vi "Three devices step test.vi"() -> ()   [LabVIEW 2015]
doc: "This example VI shows how to convert string data elements to numeric elements so it can be graphed and displayed on an XY Graph."
uses:
  <instrlib>/Keithley 27XX/Public/Configure/Measurement Specific/Configure Thermocouple.vi
  <instrlib>/Ke24xx/Ke24xx.llb/Ke24xx Configure Source Volt/Cur Level.vi
  <instrlib>/Ke24xx/Ke24xx.llb/Ke24xx Enable/Disable Source Output.vi
  <instrlib>/Keithley 27XX/Keithley 27XX.lvlib
panel:
  in  "level":dbl min=-1100.0 max=1100.0 step=1.0 format="%.2p"
  in  "Compliance":dbl=1.0 min=-1100.0 max=1100.0 step=1.0 format="%.2p"
  out "error out Cryocon":errorcluster
  out "error out 2425":errorcluster
  in  "Loop 2":bool
  in  "range":i32
  in  "function":i32(slide)
  in  "error in (no error) 2":errorcluster
  in  "reset device":u16(slide)=1
  in  "id query":u16(slide)=1
  in  "resource name":string="GPIB0::20::INSTR"
  out "Delta":dbl
  out "Variance":string
  in  "Setpoint (K)":dbl=300.0
  in  "D":sgl format="%.2f"
  in  "I":sgl=30.0 min=0 step=1 format="%.2f"
  in  "P":sgl=5.0 format="%.2f"
  in  "Output":u8(ring) items=["Loop 1", "Loop 2"]
  in  "Loop 1":bool
  out "Minimum":string
  out "Time Since Reset (Mins)":string
  out "Maximum":string
  out "Offset":string
  out "Cryocon Temp":dbl(graph)
  in  "Set Input":u8(ring) items=["ChA", "ChB", "ChC", "ChD"]
  in  "error in (no error)":errorcluster
  in  "baud rate (9600)":u32=9600
  in  "Port":string="10::INSTR"
  in  "Interface":u16(ring) items=["GPIB", "Serial"]
  in  "Save File?":bool
  out "Channel 3":dbl[](graph)
  out "Channel 2":dbl[](graph)
  out "Channel 1":dbl[](graph)
  in  "Enable Open Detector? (False)":bool
  in  "Simulated Reference Temperature (23 deg C)":dbl=23.0
  in  "Reference Junction Type (0: Simulated)":u16(ring)=1 items=["Simulated", "Internal", "External"]
  in  "Thermocouple Type (1: K)":u16(ring)=1 items=["J", "K", "T", "E", "R", "S", "B", "N"]
  in  "Column headers":string[](array[string])=["Time/s", "Cryocon Temp/C", "Ch101 Temp/C", "", "", "", ""]
  in  "Number of channels":i32=1
  in  "Pause/Continue":bool
  in  "stop":bool
  out "Iterations":i32
  out "concatenated string":string
  in  "file (use dialog)":path=path "C:/Users/Guest_2/Desktop/Zong Long/Data trial.txt"
  in  "Function (6: Temp)":u16(ring)=6 items=["DC Voltage", "AC Voltage", "DC Current", "AC Current", "Resistance", "Four-Wire Resistance", "Temperature (C)", "Frequency", "Period", "Continuity"]
  in  "Channel List (101)":string="101"
  in  "Serial Configuration":T1={"Baud Rate (9600)"=9600, "Flow Control (1: XON/XOFF)"=1, "Termination Char (0:CR)"=0} {"Termination Char (0:CR)" items=["CR", "LF", "CRLF (Do not use)", "LFCR (Do not use)"]; "Flow Control (1: XON/XOFF)" items=["None", "XON/XOFF", "RTS/CTS (2701 Only)", "XON/XOFF & RTS/CTS (2701 Only)"]; "Baud Rate (9600)" items=["300"=300, "600"=600, "1200"=1200, "2400"=2400, "4800"=4800, "9600"=9600, "19.2k"=19200, "38.4k (2701 Only)"=38400, "57.6k (2701 Only)"=57600, "115.2k (2701 Only)"=115200]}
  in  "Keithley VISA \nresource name":refnum<visa-resource-name>="GPIB0::19::INSTR"
  # "Keithley 2425 INIT"
  # "Cryocon INIT"
  # "File INIT"
  # "Keithley 2700 INIT"
  # "Operations"
  # "Only Loop 1 implemened"
  # "Data"
  # "Loop 1"
  # "Loop 2"
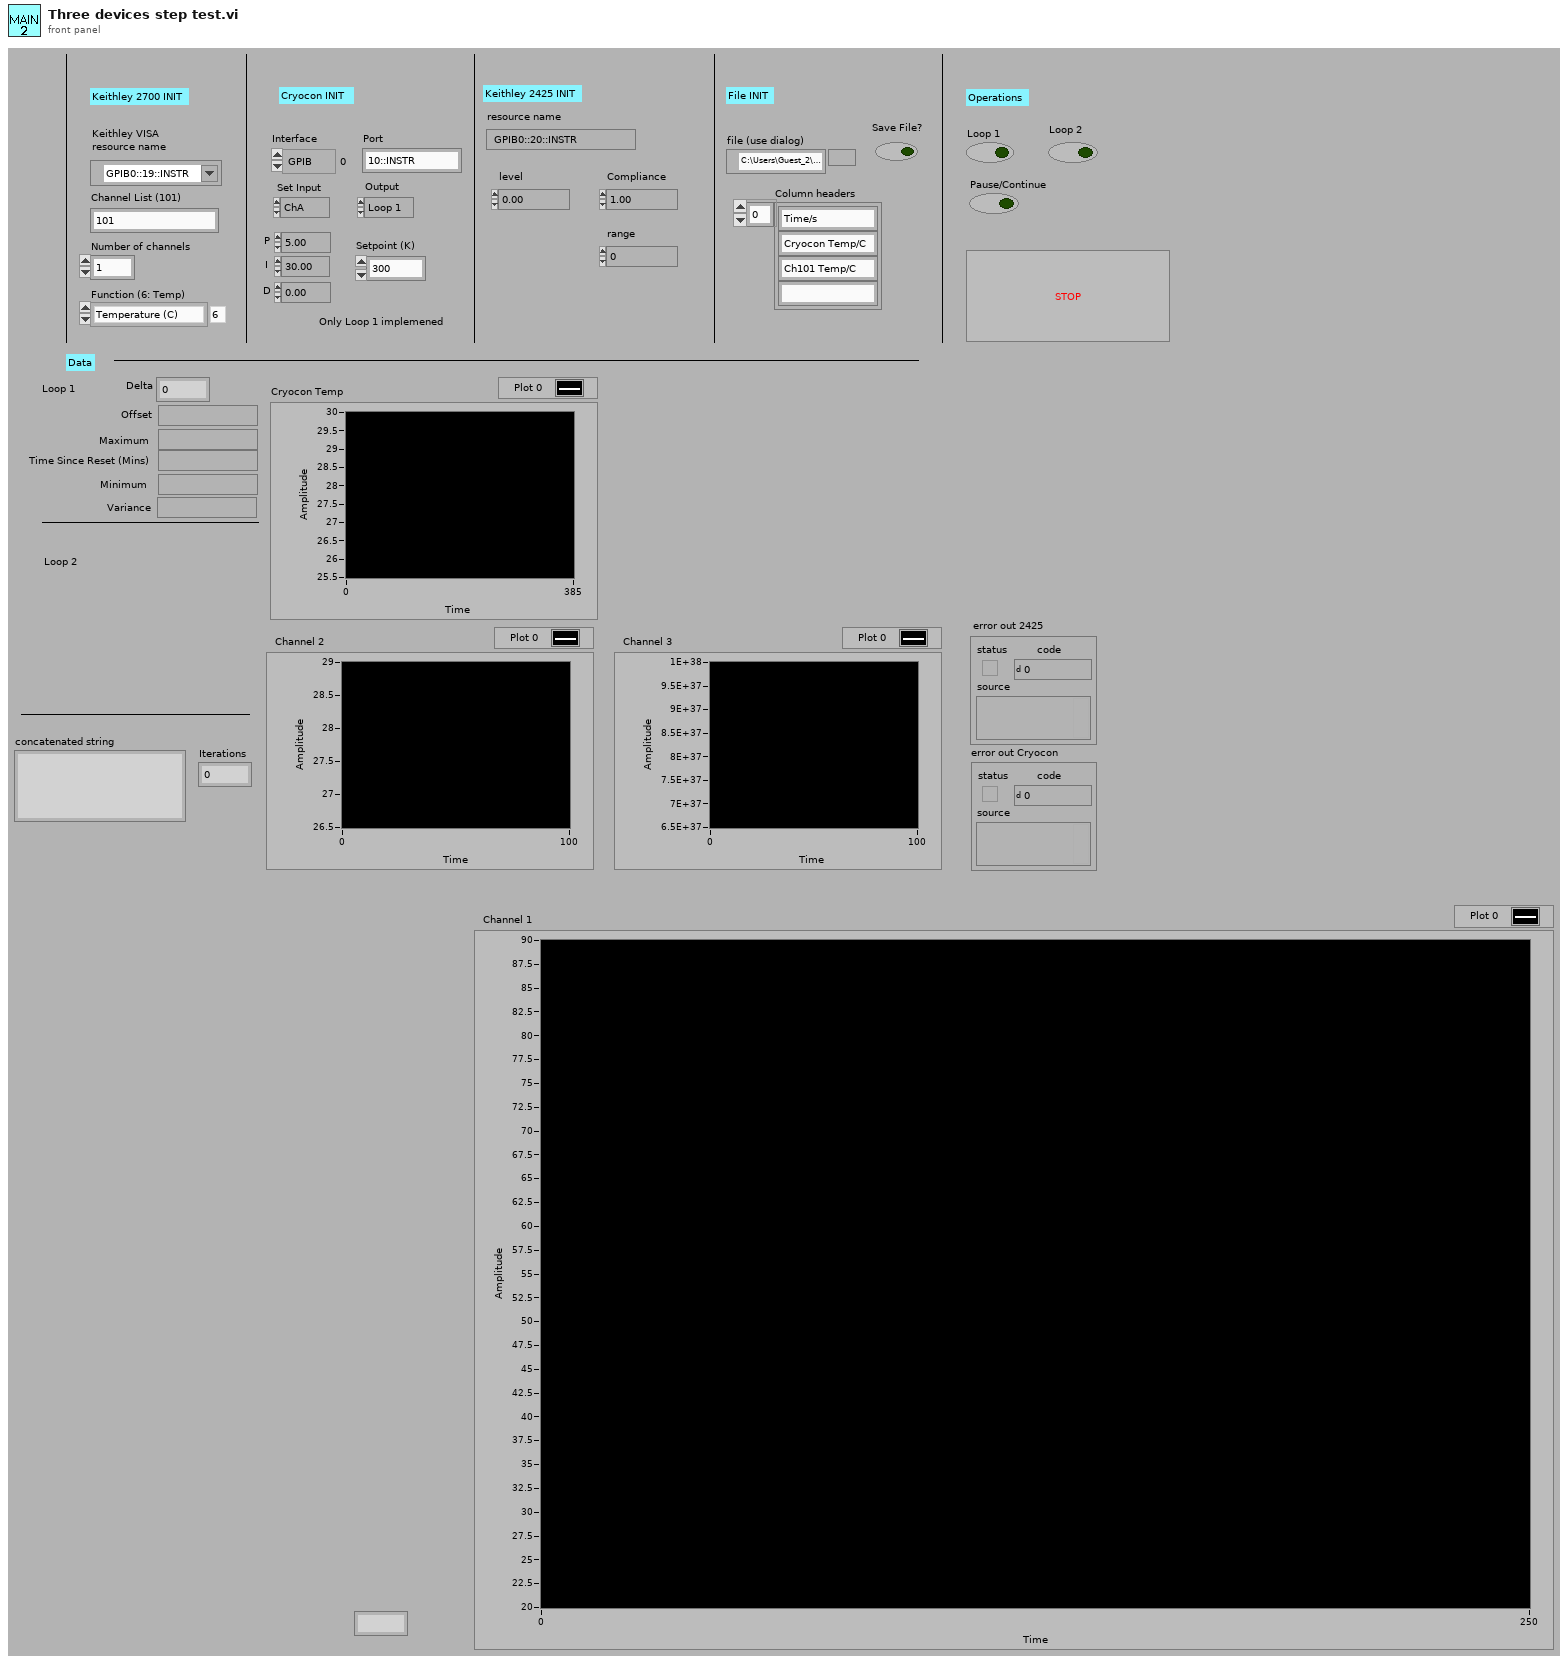
[diagram p1: front panel]
types:
  T1 = cluster{"Baud Rate (9600)":u32, "Flow Control (1: XON/XOFF)":u16, "Termination Char (0:CR)":u16}
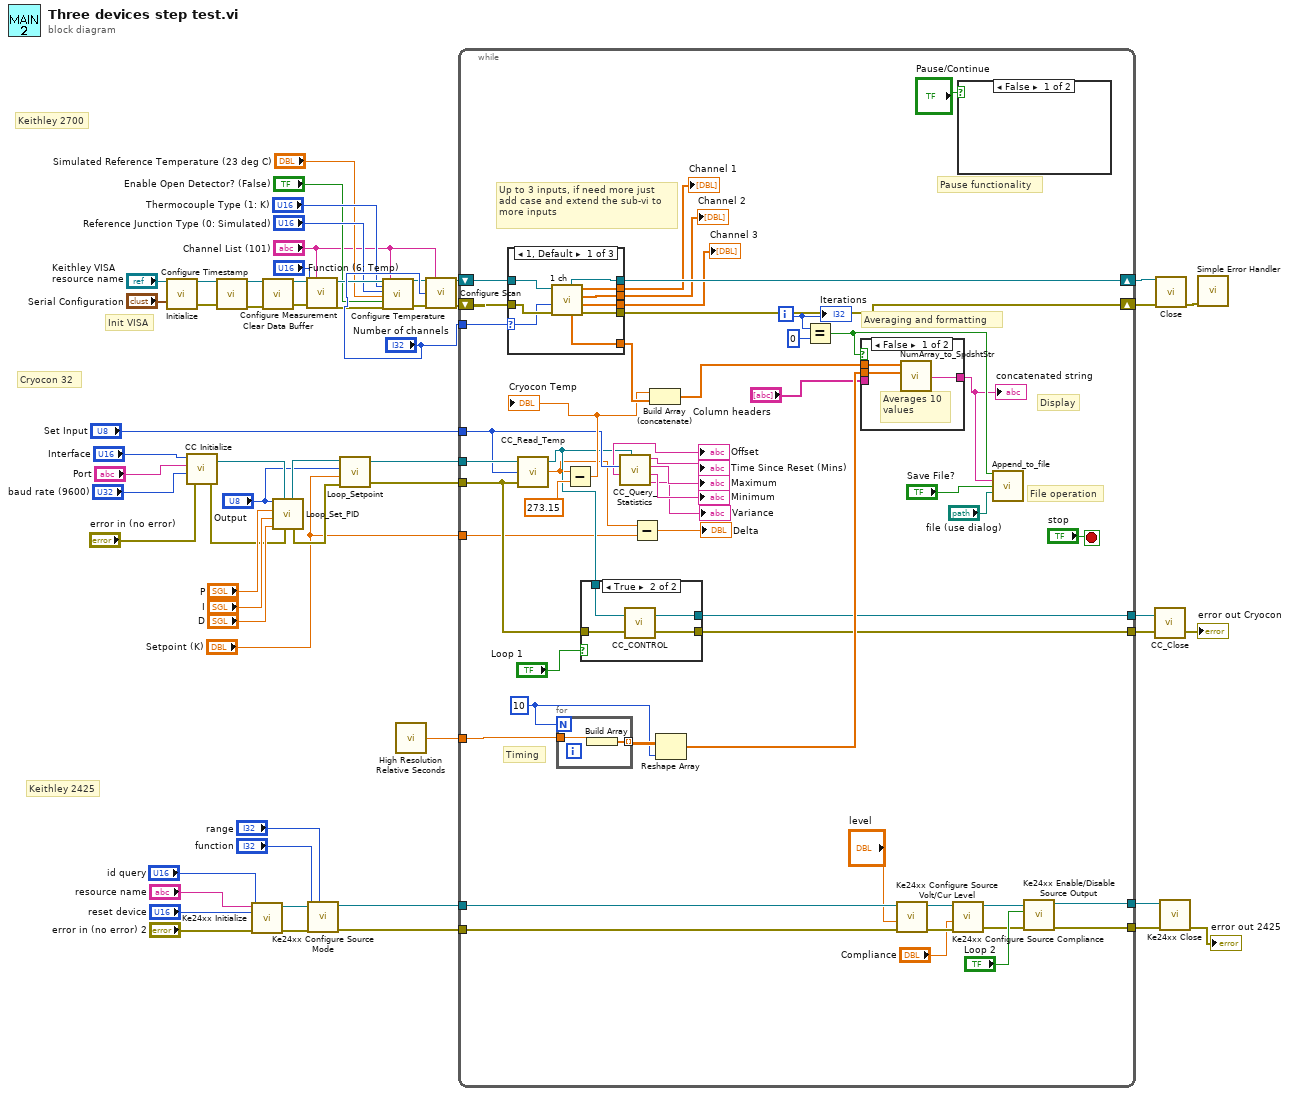
[diagram p0: block diagram]
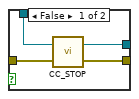
[diagram p2: hidden frame]
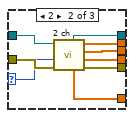
[diagram p3: hidden frame]
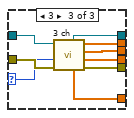
[diagram p4: hidden frame]
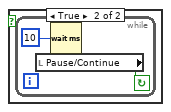
[diagram p5: hidden frame]
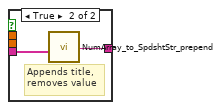
[diagram p6: hidden frame]
diagram:
  # "Keithley 2425"
  # "Cryocon 32"
  # "Keithley 2700"
  # "Init VISA"
  n1 = call <instrlib>:"Initialize.vi"("VISA resource name"="Keithley VISA \nresource name", "Serial Configuration"="Serial Configuration") -> ("VISA resource name out"=w54:refnum<visa-resource-name>, "error out"=w53:errorcluster)  [unwired: 12 in]
  n2 = call "CC Initialize.vi"("error in (no error)"="error in (no error)", "baud rate (9600)"="baud rate (9600)", "Port"="Port", "Interface"="Interface") -> ("error out"=w22:errorcluster, "VISA out"=w21:refnum<visa-resource-name>)
  n3 = call <instrlib>:"Configure Timestamp.vi"("VISA resource name"=w54, "error in (no error)"=w53) -> ("VISA resource name out"=w49:refnum<visa-resource-name>, "error out"=w48:errorcluster)  [unwired: 12 in]
  n4 = call <instrlib>:"Ke24xx Initialize.vi"("error in (no error)"="error in (no error) 2", "reset device"="reset device", "id query"="id query", "resource name"="resource name") -> ("error out"=w9:errorcluster, "instrument handle out"=w10:refnum<visa-resource-name>)  [unwired: 5 in, 1 out]
  n5 = call <instrlib>:"Clear Data Buffer.vi"("VISA resource name"=w49, "error in (no error)"=w48) -> ("VISA resource name out"=w47:refnum<visa-resource-name>, "error out"=w50:errorcluster)  [unwired: 12 in]
  n6 = call "Loop_Set_PID"("error in (no error)"=w22, "VISA In"=w21, "D"="D", "I"="I", "P"="P", "Output"="Output") -> ("error out"=w20:errorcluster, "VISA Out"=w19:refnum<visa-resource-name>)  [unwired: 4 in]
  n7 = call <instrlib>:"Configure Measurement.vi"("VISA resource name"=w47, "Scan List (Empty)"="Channel List (101)", "Function (0: DC Voltage)"="Function (6: Temp)", "error in (no error)"=w50) -> ("VISA resource name out"=w41:refnum<visa-resource-name>, "error out"=w38:errorcluster)  [unwired: 10 in]
  n8 = call <instrlib>:"Ke24xx Configure Source Mode.vi"("range"="range", "error in (no error)"=w9, "function"="function", "instrument handle"=w10) -> ("error out"=w1:errorcluster, "instrument handle out"=w2:refnum<visa-resource-name>)  [unwired: 5 in, 1 out]
  n9 = call "Loop_Setpoint.vi"("VISA in"=w19, "Loop"="Output", "Setpoint"="Setpoint (K)", "error in"=w20) -> ("VISA out"=w18:refnum<visa-resource-name>, "ErrorOut"=w16:errorcluster)  [unwired: 1 in, 1 out]
  n10 = call-poly <instrlib>:"Configure Temperature.vi"("VISA resource name"=w41, "Thermocouple Type (1: K)"="Thermocouple Type (1: K)", "Reference Junction Type (0: Simulated)"="Reference Junction Type (0: Simulated)", "Simulated Reference Temperature (23 deg C)"="Simulated Reference Temperature (23 deg C)", "Enable Open Detector? (False)"="Enable Open Detector? (False)", "error in (no error)"=w38, "Scan List (Empty)"="Channel List (101)") -> ("VISA resource name out"=w40:refnum<visa-resource-name>, "error out"=w39:errorcluster)  [unwired: 11 in]
  n11 = call <vilib>:"High Resolution Relative Seconds.vi"() -> ("relative seconds"=w43:dbl)
  n12 = call <instrlib>:"Configure Scan.vi"("VISA resource name"=w40, "Channel List (101:110)"="Channel List (101)", "Sample Count (100)"="Number of channels", "error in (no error)"=w39) -> ("VISA resource name out"=w45:refnum<visa-resource-name>, "error out"=w44:errorcluster)  [unwired: 10 in]
  n13 = while {
    shift-right: [w107] -> w51
    shift-left: w45 -> [w106]
    shift-right: [w108] -> w52
    shift-left: w44 -> [w105]
    tunnel: w43 -> [w103]
    tunnel: "Number of channels" -> [w96]
    tunnel: "Set Input" -> [w83]
    tunnel: w18 -> [w88]
    tunnel: w16 -> [w76]
    tunnel: [w75] -> w27
    tunnel: [w74] -> w26
    tunnel: "Setpoint (K)" -> [w71]
    tunnel: [w68] -> w6
    tunnel: [w67] -> w5
    tunnel: w2 -> [w66]
    tunnel: w1 -> [w65]
    i -> [w98]
    stop <- "stop" stop-if-true
    w95 = 10 ("x")
    # "Timing"
    # "Up to 3 inputs, if need more just\nadd case and extend the sub-vi to\nmore inputs"
    # "Display"
    # "Averaging and formatting"
    # "File operation"
    # "Pause functionality"
    n14 = case shown="1, Default" w96 {
      selector: w96 -> [w124 w131 w140]
      tunnel: [w120 w132 w141] -> w108
      tunnel: [w122 w129 w139] -> w107
      tunnel: w106 -> [w123 w134 w142]
      tunnel: w105 -> [w125 w133 w143]
      tunnel: [w119 w127 w137] -> w59
      tunnel: [w118 w128 w136] -> w94
      tunnel: [w117 w130 w135] -> w93
      tunnel: [w121 w126 w138] -> w86
      frame 1, Default {
        n15 = call "1 ch.vi"("error out"=w125, "Number of channels"=w124, "VISA resource name out"=w123) -> ("error out 2"=w120:errorcluster, "output array 3"=w117:dbl[], "output array 2"=w118:dbl[], "Means of 10"=w119:dbl[], "output array"=w121:dbl[], "VISA resource name out 2"=w122:refnum<visa-resource-name>)  [unwired: 3 in]
      }
      frame 2 {
        n16 = call "2 ch.vi"("error out"=w133, "Number of channels"=w131, "VISA resource name out"=w134) -> ("error out 2"=w132:errorcluster, "Means of 12"=w130:dbl[], "Means of 11"=w128:dbl[], "Means of 10"=w127:dbl[], "output array"=w126:dbl[], "VISA resource name out 2"=w129:refnum<visa-resource-name>)  [unwired: 3 in]
      }
      frame 3 {
        n17 = call "3 ch.vi"("error out"=w143, "Number of channels"=w140, "VISA resource name out"=w142) -> ("error out 2"=w141:errorcluster, "Means of 12"=w135:dbl[], "Means of 11"=w136:dbl[], "Means of 10"=w137:dbl[], "output array"=w138:dbl[], "VISA resource name out 2"=w139:refnum<visa-resource-name>)  [unwired: 3 in]
      }
    }
    "Channel 3" <- w93
    "Channel 2" <- w94
    "Channel 1" <- w59
    n18 = call "CC_Read_Temp.vi"("error in (no error)"=w76, "Input"=w83, "VISA In"=w88) -> ("Temperature"=w72:dbl, "VISA Out"=w77:refnum<visa-resource-name>)  [unwired: 1 out]
    n19 = for {
      N: w95 -> [_]
      tunnel: w103 -> [w147]
      tunnel: [w146] -> w102 mode=indexing
      n20 = Build Array(w147) -> (w146:dbl[])
    }
    n21 = Subtract(x=w72, y=273.15) -> (x-y=w84:dbl)
    "Cryocon Temp" <- w84
    n22 = case shown="True" "Loop 1" {
      tunnel: w77 -> [w112 w116]
      tunnel: w76 -> [w111 w115]
      tunnel: [w110 w114] -> w75
      tunnel: [w109 w113] -> w74
      frame False {
        n23 = call "CC_STOP.vi"("error in (no error)"=w111, "VISA In"=w112) -> ("error out"=w109:errorcluster, "VISA Out"=w110:refnum<visa-resource-name>)
      }
      frame True {
        n24 = call "CC_CONTROL.vi"("error in (no error)"=w115, "VISA In"=w116) -> ("error out"=w113:errorcluster, "VISA Out"=w114:refnum<visa-resource-name>)
      }
    }
    n25 = call "CC_Query_Statistics.vi"("VISA In"=w77, "Input"=w83) -> ("Variance"=→"Variance":string, "Minimum"=→"Minimum":string, "Maximum"=→"Maximum":string, "Time Since Reset"=→"Time Since Reset (Mins)":string, "Offset"=→"Offset":string)  [unwired: 2 in, 3 out]
    n26 = Subtract(x=w72, y=w71) -> (x-y=→"Delta":dbl)
    n27 = Build Array (concatenate)(w84, w86) -> (w87:dbl[])
    n28 = Reshape Array(w102, w95) -> (w101:dbl[])
    n29 = Equal?(x=w98, y=0) -> (x = y?=w91:bool)
    n30 = case shown="False" w91 {
      tunnel: w87 -> [w150 _]
      tunnel: w101 -> [w149 _]
      tunnel: [w148 w152] -> w90
      tunnel: "Column headers" -> [_ w151]
      frame False {
        # "Averages 10 \nvalues"
        n31 = call "NumArray_to_SpdshtStr.vi"("element 2"=w149, "element"=w150) -> ("concatenated string"=w148:string)  [unwired: 8 in, 1 out]
      }
      frame True {
        # "Appends title,\nremoves value"
        n32 = call "NumArray_to_SpdshtStr_prepend.vi"("Column headers"=w151) -> ("concatenated string"=w152:string)  [unwired: 10 in]
      }
    }
    "concatenated string" <- w90
    n33 = call "Ke24xx Configure Source Volt/Cur Level.vi"("error in (no error)"=w65, "level"="level", "instrument handle"=w66) -> ("error out"=w63:errorcluster, "instrument handle out"=w64:refnum<visa-resource-name>)  [unwired: 6 in, 1 out]
    n34 = call <instrlib>:"Ke24xx Configure Source Compliance.vi"("error in (no error)"=w63, "level"="Compliance", "instrument handle"=w64) -> ("error out"=w61:errorcluster, "instrument handle out"=w62:refnum<visa-resource-name>)  [unwired: 6 in, 1 out]
    n35 = case shown="False" "Pause/Continue" {
      frame False {
      }
      frame True {
        n36 = while {
          stop <- w145 continue-if-true
          n37 = local read "Pause/Continue"() -> (w145:bool)
          n38 = Wait (ms)(milliseconds to wait=u32 10) -> ()  [unwired: 1 out]
        }
      }
    }
    n39 = call "Append_to_file.vi"("Boolean"=w91, "text"=w90, "Save File?"="Save File?", "file path (use dialog)"="file (use dialog)") -> ()  [unwired: 11 in, 1 out]
    n40 = call "Ke24xx Enable/Disable Source Output.vi"("error in (no error)"=w61, "state"="Loop 2", "instrument handle"=w62) -> ("error out"=w67:errorcluster, "instrument handle out"=w68:refnum<visa-resource-name>)  [unwired: 6 in, 1 out]
    "Iterations" <- w98
  }
  n41 = call "CC_Close.vi"("error in (no error)"=w26, "VISA In"=w27) -> ("error out"=→"error out Cryocon":errorcluster)  [unwired: 1 in]
  n42 = call <instrlib>:"Close.vi"("VISA resource name"=w51, "error in (no error)"=w52) -> ("error out"=w55:errorcluster)  [unwired: 13 in]
  n43 = call <instrlib>:"Ke24xx Close.vi"("error in (no error)"=w5, "instrument handle"=w6) -> ("error out"=→"error out 2425":errorcluster)  [unwired: 8 in, 1 out]
  n44 = call <vilib>:"Simple Error Handler.vi"("error in (no error)"=w55) -> ()  [unwired: 4 in, 5 out]
